vi "SP Convert Measurements Cluster.vi"(4 "Conversion":enum16{"Cluster - HTML", "HTML - Cluster"}(ring), 6 "Measurements Key Array In":T4, 7 "Measurements Cluster In":T1={"Auto Select"=TRUE, "Data Source"=enum."VNA", "Ports"=2, "Parameters"=[]} {"Parameters"."Channel" min=0 max=32 step=1; "Parameters"."Parameter"."Stimulus Port" min=1 step=1; "Parameters"."Parameter"."Response Port" min=1 step=1}) -> (1 "Measurements Cluster Out":T1={"Auto Select"=TRUE, "Data Source"=enum."VNA", "Ports"=2, "Parameters"=[]} {"Parameters"."Channel" min=0 max=32 step=1; "Parameters"."Parameter"."Stimulus Port" min=1 step=1; "Parameters"."Parameter"."Response Port" min=1 step=1}, 2 "Measurements HTML Out":string)   [LabVIEW 2011]
uses:
  ITK/utils/keyedarr.llb/Keyed Array.ctl
  TypeDefs/SP Measurement.ctl
  TypeDefs/SP Parameters.ctl
  TypeDefs/SP Parameter.ctl
  ITK/utils/strutil.llb/Case Matching.ctl
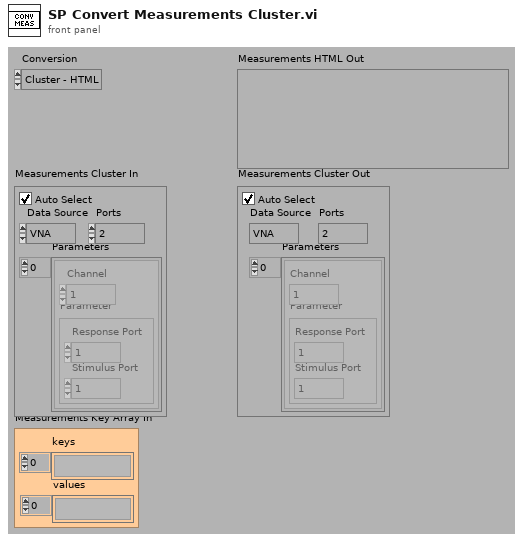
[diagram p1: front panel]
types:
  T1 = typedef "SP Measurement.ctl" = cluster{"Auto Select":bool, "Data Source":enum16{"VNA", "Data File"}, "Ports":i8, "Parameters":T2[]}
  T2 = typedef "SP Parameters.ctl" = cluster{"Channel":i8, "Parameter":T3}
  T3 = typedef "SP Parameter.ctl" = cluster{"Stimulus Port":i8, "Response Port":i8}
  T4 = typedef "Keyed Array.ctl" = cluster{"keys":string[], "values":string[]}
  T5 = typedef "Case Matching.ctl" = enum16{"a != A", "a == A", "system"}
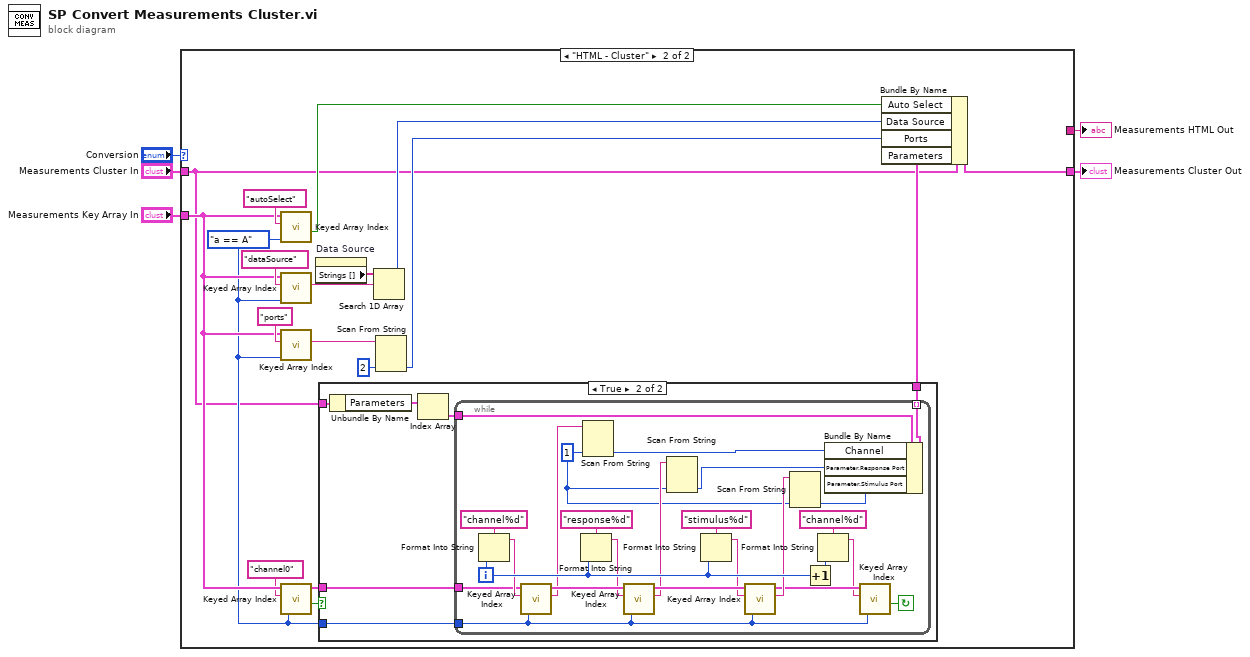
[diagram p0: block diagram]
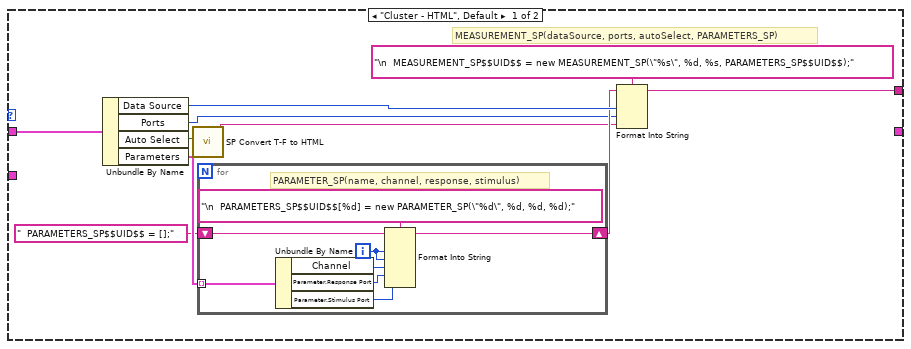
[diagram p2: hidden frame]
diagram:
  n1 = case shown="\"HTML - Cluster\"" "Conversion" {
    tunnel: "Measurements Cluster In" -> [w15 w24]
    tunnel: "Measurements Key Array In" -> [_ w29]
    tunnel: [w10 _] -> w2
    tunnel: [_ w35] -> w1
    frame "Cluster - HTML", Default {
      # "MEASUREMENT_SP(dataSource, ports, autoSelect, PARAMETERS_SP)"
      n2 = Unbundle By Name(w15) -> ("Data Source"=w9:enum16{"VNA", "Data File"}, "Ports"=w7:i8, "Auto Select"=w13:bool, "Parameters"=w12:T2[])
      n3 = call "SP Convert T-F to HTML.vi"("(T/F)"=w13) -> ("HTML (true/false)"=w6:string)  [unwired: 10 out]
      n4 = for {
        tunnel: w12 -> [w23] mode=indexing
        shift-right: [w18] -> w8
        shift-left: "  PARAMETERS_SP$$UID$$ = [];" ("format string") -> [w17]
        i -> [w16]
        # "PARAMETER_SP(name, channel, response, stimulus)"
        n5 = Unbundle By Name(w23) -> ("Channel"=w20:i8, "Parameter.Response Port"=w19:i8, "Parameter.Stimulus Port"=w21:i8)
        n6 = Format Into String(format string="\n  PARAMETERS_SP$$UID$$[%d] = new PARAMETER_SP(\"%d\", %d, %d, %d);", initial string=w17, w16, w16, w20, w19, w21) -> (resulting string=w18:string)  [unwired: 1 in, 1 out]
      }
      n7 = Format Into String(format string="\n  MEASUREMENT_SP$$UID$$ = new MEASUREMENT_SP(\"%s\", %d, %s, PARAMETERS_SP$$UID$$);", initial string=w8, w9, w7, w6) -> (resulting string=w10:string)  [unwired: 1 in, 1 out]
    }
    frame "HTML - Cluster" {
      w28 = Case_Matching."a == A" ("case matching (sensitive)")
      n8 = call "Keyed Array Index.vi"("case matching (sensitive)"=w28, "key"="autoSelect", "array in"=w29) -> ("valid key"=w38:bool)  [unwired: 1 in, 3 out]
      n9 = call "Keyed Array Index.vi"("case matching (sensitive)"=w28, "key"="dataSource", "array in"=w29) -> ("value"=w31:string)  [unwired: 1 in, 3 out]
      n10 = call "Keyed Array Index.vi"("case matching (sensitive)"=w28, "key"="ports", "array in"=w29) -> ("value"=w39:string)  [unwired: 1 in, 3 out]
      n11 = call "Keyed Array Index.vi"("case matching (sensitive)"=w28, "key"="channel0", "array in"=w29) -> ("valid key"=w25:bool, "duplicate array"=w27:T4)  [unwired: 1 in, 2 out]
      n12 = property on="Data Source" class="Enum (strict)"() -> ("Strings []"=w32:string[])  [unwired: 2 in, 2 out]
      n13 = case shown="True" w25 {
        tunnel: [_ w45] -> w36
        tunnel: w28 -> [_ w44]
        tunnel: w27 -> [_ w43]
        tunnel: w24 -> [_ w42]
        frame False {
        }
        frame True {
          n14 = Unbundle By Name(w42) -> ("Parameters"=w47:T2[])
          n15 = Index Array(array=w47) -> (element=w46:T2)  [unwired: 1 in]
          n16 = while {
            tunnel: w46 -> [w69]
            tunnel: [w68] -> w45 mode=indexing
            tunnel: w44 -> [w49]
            tunnel: w43 -> [w48]
            i -> [w72]
            stop <- w50 continue-if-true
            w55 = i8 1 ("default value 1")
            n17 = Format Into String(format string="channel%d", w72) -> (resulting string=w66:string)  [unwired: 2 in, 1 out]
            n18 = call "Keyed Array Index.vi"("case matching (sensitive)"=w49, "key"=w66, "array in"=w48) -> ("value"=w65:string, "duplicate array"=w70:T4)  [unwired: 1 in, 2 out]
            n19 = Format Into String(format string="response%d", w72) -> (resulting string=w61:string)  [unwired: 2 in, 1 out]
            n20 = Scan From String(input string=w65, default 1=w55) -> (output 1=w64:i8)  [unwired: 3 in, 3 out]
            n21 = call "Keyed Array Index.vi"("case matching (sensitive)"=w49, "key"=w61, "array in"=w70) -> ("value"=w59:string, "duplicate array"=w71:T4)  [unwired: 1 in, 2 out]
            n22 = Scan From String(input string=w59, default 1=w55) -> (output 1=w58:i8)  [unwired: 3 in, 3 out]
            n23 = Format Into String(format string="stimulus%d", w72) -> (resulting string=w60:string)  [unwired: 2 in, 1 out]
            n24 = call "Keyed Array Index.vi"("case matching (sensitive)"=w49, "key"=w60, "array in"=w71) -> ("value"=w56:string, "duplicate array"=w52:T4)  [unwired: 1 in, 2 out]
            n25 = Scan From String(input string=w56, default 1=w55) -> (output 1=w57:i8)  [unwired: 3 in, 3 out]
            n26 = Increment(x=w72) -> (x+1=w53:i32)
            n27 = Format Into String(format string="channel%d", w53) -> (resulting string=w51:string)  [unwired: 2 in, 1 out]
            n28 = Bundle By Name(cluster=w69, "Channel"=w64, "Parameter.Response Port"=w58, "Parameter.Stimulus Port"=w57) -> (w68:T2)
            n29 = call "Keyed Array Index.vi"("case matching (sensitive)"=w49, "key"=w51, "array in"=w52) -> ("valid key"=w50:bool)  [unwired: 1 in, 3 out]
          }
        }
      }
      n30 = Search 1D Array(1D array=w32, element=w31) -> (index of element=w30:i32)  [unwired: 1 out]
      n31 = Scan From String(input string=w39, default 1=i8 2 ("default value 1")) -> (output 1=w34:i8)  [unwired: 3 in, 3 out]
      n32 = Bundle By Name(cluster=w24, "Auto Select"=w38, "Data Source"=w30, "Ports"=w34, "Parameters"=w36) -> (w35:T1)
    }
  }
  "Measurements HTML Out" <- w2
  "Measurements Cluster Out" <- w1
